vi "Two Lockins.vi"(8 "error in (no error)":errorcluster, 11 "Two lockins reader in":refnum<class "Two lockins reader.lvclass">) -> (0 "error out":errorcluster, 3 "Two lockins reader out":refnum<class "Two lockins reader.lvclass">)   [LabVIEW 2017, in "Two lockins reader.lvclass"]
uses:
  Two lockins reader.lvclass
  Two lockins reader.lvclass/Two lockins reader.ctl
  Instruments/Lockin/Lockin SR830.lvclass
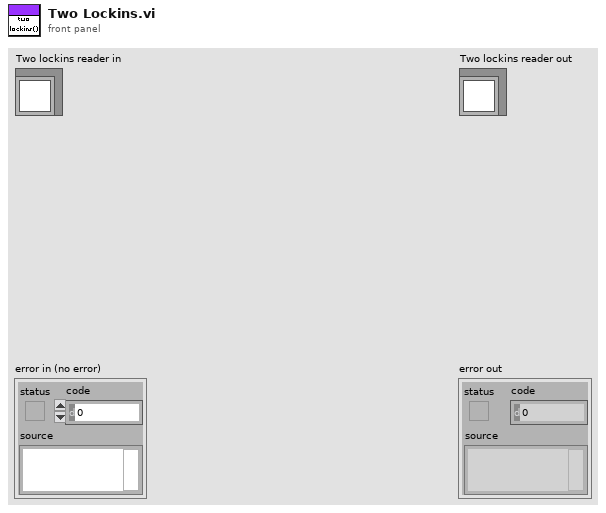
[diagram p1: front panel]
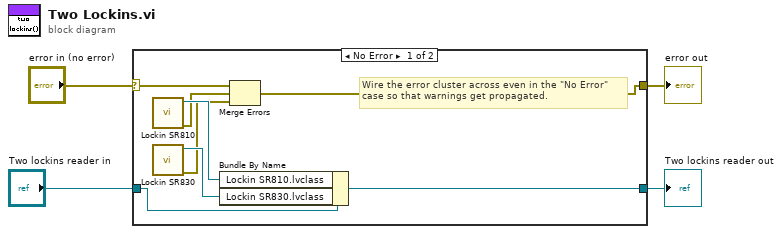
[diagram p0: block diagram]
diagram:
  n1 = case shown="No Error" "error in (no error)" {
    selector: "error in (no error)" -> [w6 w14]
    tunnel: [w5 w14] -> w3
    tunnel: [w11 w13] -> w1
    tunnel: "Two lockins reader in" -> [w12 w13]
    frame No Error {
      # "Wire the error cluster across even in the \"No Error\"\ncase so that warnings get propagated."
      n2 = call "Lockin SR810.vi"() -> ("error out"=w8:errorcluster, "Lockin SR830 out"=w10:refnum<class "Lockin SR830.lvclass">)  [unwired: 10 in]
      n3 = call "Lockin SR830.vi"() -> ("error out"=w7:errorcluster, "Lockin SR830 out"=w9:refnum<class "Lockin SR830.lvclass">)  [unwired: 10 in]
      n4 = Bundle By Name(cluster=w12, "Lockin SR810.lvclass"=w10, "Lockin SR830.lvclass"=w9) -> (w11:refnum<class "Two lockins reader.lvclass">)
      n5 = Merge Errors(w6, w8, w7) -> (w5:errorcluster)
    }
    frame Error {
    }
  }
  "error out" <- w3
  "Two lockins reader out" <- w1
